vi "execute and fetch.vi"(8 "error in (no error)":errorcluster, 10 "SQL query":string, 11 "Database in":refnum<class "Database.lvclass">) -> (0 "error out":errorcluster, 1 "Num records":i32, 2 "recordset data":variant[][](array[variant]), 3 "Database out":refnum<class "Database.lvclass">)   [LabVIEW 2018, in "Database.lvclass"]
uses:
  Database.lvclass
  Database.lvclass/Database.ctl
  <vilib>/addons/database/Connection.llb/Conn Execute.vi
  <vilib>/addons/database/Recordset.llb/Rec Fetch Recordset Data (R).vi
  <vilib>/addons/database/Recordset.llb/Rec Destroy - Connection.vi
  <vilib>/addons/database/NI_Database_API.lvlib
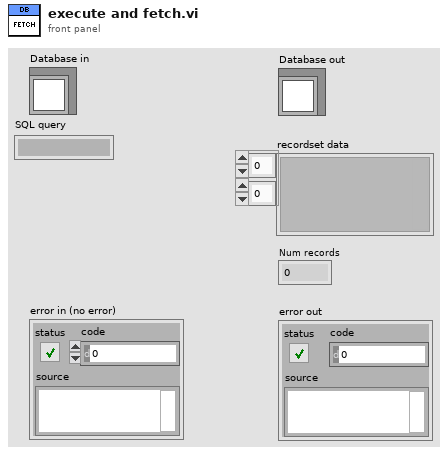
[diagram p1: front panel]
types:
  T1 = typedef "NI_Database_API.lvlib/Conn ObjectReference.ctl" = refnum<k1>
  T2 = typedef "NI_Database_API.lvlib/Rec ObjectReference.ctl" = refnum<k1>
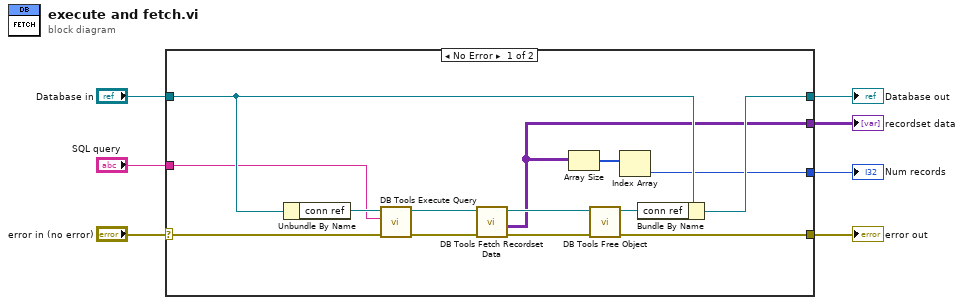
[diagram p0: block diagram]
diagram:
  n1 = case shown="No Error" "error in (no error)" {
    selector: "error in (no error)" -> [w12 w22]
    tunnel: [w21 w22] -> w7
    tunnel: [w20 w23] -> w6
    tunnel: "Database in" -> [w18 w23]
    tunnel: [w9 _] -> w4
    tunnel: "SQL query" -> [w11 _]
    tunnel: [w8 _] -> w1
    frame No Error {
      n2 = Unbundle By Name(w18) -> ("conn ref"=w17:T1)
      n3 = call-poly <vilib>:"DB Tools Execute Query.vi"("error in (no error)"=w12, "SQL query"=w11, "connection reference"=w17) -> ("error out"=w15:errorcluster, "recordset reference"=w16:T2)  [unwired: 2 in, 3 out]
      n4 = call-poly <vilib>:"DB Tools Fetch Recordset Data.vi"("error in (no error)"=w15, "recordset reference"=w16) -> ("error out"=w13:errorcluster, "recordset data"=w9:variant[][], "recordset reference out"=w14:T2)  [unwired: 3 out]
      n5 = Array Size(array=w9) -> (size(s)=w10:i32[])
      n6 = call-poly <vilib>:"DB Tools Free Object.vi"("error in (no error)"=w13, "recordset reference"=w14) -> ("error out"=w21:errorcluster, "connection reference"=w19:T1)  [unwired: 8 out]
      n7 = Index Array(array=w10) -> (element=w8:i32)  [unwired: 1 in]
      n8 = Bundle By Name(cluster=w18, "conn ref"=w19) -> (w20:refnum<class "Database.lvclass">)
    }
    frame Error {
    }
  }
  "error out" <- w7
  "Database out" <- w6
  "recordset data" <- w4
  "Num records" <- w1
